vi "Check Version.vi"(8 "error in (no error)":errorcluster, 11 "LV Argument Parser in":refnum<class "LV Argument Parser.lvclass">) -> (0 "error out":errorcluster, 2 "Output":string, 3 "LV Argument Parser out":refnum<class "LV Argument Parser.lvclass">)   [LabVIEW 2023, in "LV ArgParse.lvlib" / "LV Argument Parser.lvclass"]
uses:
  LV Argument Parser.lvclass
  LV Argument Parser.lvclass/LV Argument Parser.ctl
  LV ArgParse.lvlib
  Get Bool.vi
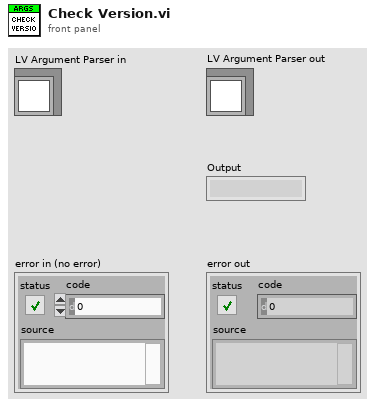
[diagram p1: front panel]
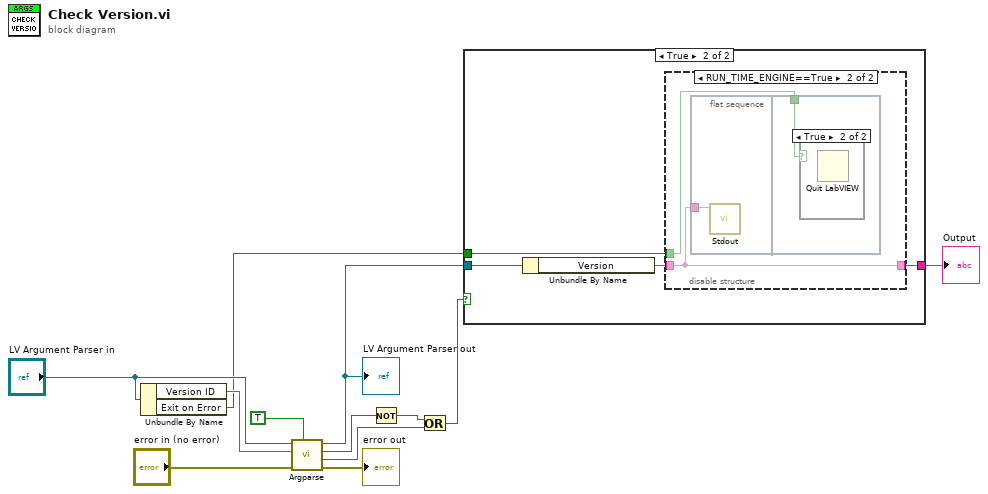
[diagram p0: block diagram]
diagram:
  n1 = Unbundle By Name("LV Argument Parser in") -> ("Version ID"=w8:string, "Exit on Error"=w1:bool)
  n2 = call-poly "Argparse.vi"("Optional"=TRUE, "error in (no error)"="error in (no error)", "Name"=w8, "LV Argument Parser in"="LV Argument Parser in") -> ("error out"=→"error out":errorcluster, "Value"=w5:bool, "key not found?"=w3:bool, "LV Argument Parser out"=w6:refnum<class "LV Argument Parser.lvclass">)  [unwired: 4 in]
  "LV Argument Parser out" <- w6
  n3 = Not(x=w3) -> (.not. x?=w4:bool)
  n4 = Or(x=w4, y=w5) -> (x .or. y?=w2:bool)
  n5 = case shown="True" w2 {
    tunnel: w6 -> [_ w16]
    tunnel: [_ w14] -> w12
    tunnel: w1 -> [_ w13]
    frame False {
    }
    frame True {
      n6 = Unbundle By Name(w16) -> ("Version"=w15:string)
      n7 = disable-structure shown="RUN_TIME_ENGINE==True" {
        disable-tunnel: w15 -> [w17 w18]
        disable-tunnel: [w17 w18] -> w14
        disable-tunnel: w13 -> [_ w19]
        frame condition #0 (active) {
        }
        frame condition #1 {
          n8 = flat-sequence {
            tunnel: w18 -> [w20]
            tunnel: w19 -> [w21]
            frame #0 {
              n9 = call "Stdout.vi"("text"=w20) -> ()  [unwired: 10 in, 1 out]
            }
            frame #1 {
              n10 = case shown="True" w21 {
                frame False {
                }
                frame True {
                  n11 = Quit LabVIEW() -> ()  [unwired: 1 in]
                }
              }
            }
          }
        }
      }
    }
  }
  "Output" <- w12
